vi "save expt configuration to database.vi"(8 "error in (no error)":errorcluster, 9 "configuration name":string, 10 "experiment name":string, 11 "Device Name":string) -> (0 "error out":errorcluster)   [LabVIEW 2020]
uses:
  Shared/MySQL/Preset Query Enum.ctl
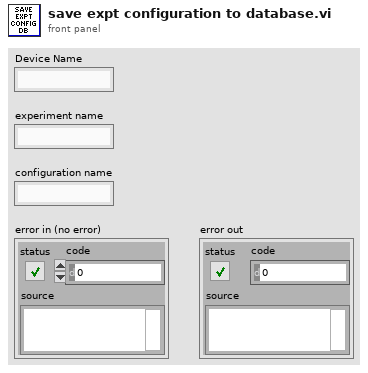
[diagram p1: front panel]
types:
  T1 = typedef "Preset Query Enum.ctl" = enum16{"Get Locations", "Get all IPs and MACs", "Get classes", "Get expt variables to set at scanstart for particular device", "Get expt devices and variables with start values", "Get expt devices and variables (with data to get)", "Get expt devices with data to get", "Get Expt devices and GUIs", "Get all devices basic properties", "Get Virtual Devices Core Info", "Get Expt names", "Get experiment basic properties", "Get experiment alarm variables", "Get MC Ports", "Get device network comm port", "Get devicetype lvclass path", "Get basic device properties", "Get Init Order", "Get all setable variables of a device", "Get device variable aliases", "Get force values of all settable variables", "Get all variables of a devicetype", "Get all variables of a device", "Get plotter details", "Get Saved Scans", "Get Scan Info", "GetGeneralGUIs", "Get expt for plotter", "Get plotter IDs from expt", "Get all devices", "Get all Virtual Devices", "Get all aliases", "Get variable and device info for Virtual Device", "GetItemLocatorIP", "Get IPs for GUIs", "Get DeviceType from Device", "GetLocalPortRange", "GetDevicePresetVariables", "Get Device Configuration", "GetAllPresetNames", "GetAllConfigurationNames", "GetPresetDeviceNames"}
  T2 = typedef "mysql_authentication.ctl" = cluster{"User":string, "Password":string, "Database":string}
  T3 = cluster{"Port":u16, "IP Address":string, "Authentication":T2}
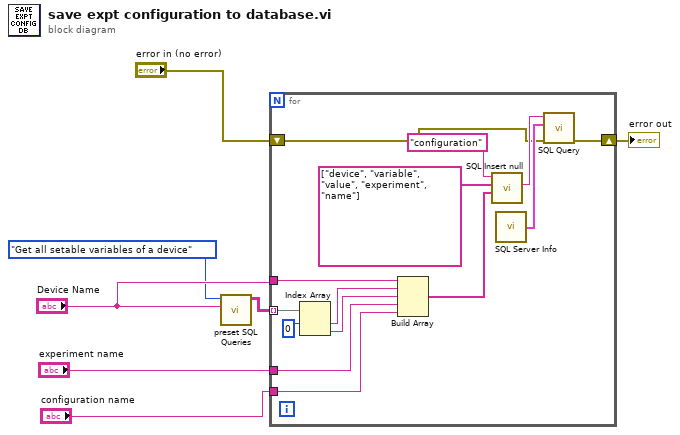
[diagram p0: block diagram]
diagram:
  n1 = call "preset SQL Queries.vi"("Device/Devicetype name\n/Plotter.id/ScanName#"="Device Name", "Preset Query"=Preset_Query_Enum."Get all setable variables of a device") -> ("data"=w2:string[][])  [unwired: 7 in, 2 out]
  n2 = for {
    tunnel: w2 -> [w15] mode=indexing
    shift-right: [w11] -> w4
    shift-left: "error in (no error)" -> [w12]
    tunnel: "configuration name" -> [w10]
    tunnel: "experiment name" -> [w9]
    tunnel: "Device Name" -> [w8]
    n3 = Index Array(array=w15, index #1=0 ("index")) -> (element #1=w14:string, element #2=w13:string)  [unwired: 1 in]
    n4 = Build Array(w8, w14, w13, w9, w10) -> (w17:string[])
    n5 = call "SQL Insert null.vi"("Values"=w17, "Column Names"=string[] ["device", "variable", "value", "experiment", "name"], "Table"="configuration") -> ("Query String"=w20:string)  [unwired: 8 in]
    n6 = call "SQL Server Info.vi"() -> ("SQL Server Info"=w21:T3)
    n7 = call "SQL Query.vi"("error in (no error)"=w12, "SQL Server Info"=w21, "Query"=w20) -> ("error out"=w11:errorcluster)  [unwired: 7 in, 1 out]
  }
  "error out" <- w4
